vi "Actor Core.vi"(8 "error in":errorcluster, 11 "Measure-Pulse in":refnum<class "Monitor-Pulse.lvclass">) -> (0 "error out":errorcluster, 3 "Actor out":refnum<class "Actor.lvclass">)   [LabVIEW 2016, in "Monitor-Pulse.lvclass"]
doc: "(<B>Filename</B>: Actor Framework.lvlib:Actor.lvclass:Actor Core.vi)\n\nReceives messages to the actor, reacts to them, and initiates any error handling that may shut the actor down.\n\nDescendant classes may override this VI to append parallel tasks for the actor to complete while it handles messages. Overrides use the Call Parent Method node."
uses:
  Monitor-Pulse.lvclass
  C:/github/LabActor/Controllers/Application Controller/Application Controller.lvclass
  C:/github/LabActor/Template Module/Template Module.lvclass
  C:/Program Files/National Instruments/LabVIEW 2016/vi.lib/ActorFramework/Actor/Actor.lvclass
  <vilib>/ActorFramework/Actor/Actor.lvclass
  NHMFL_Core/Libraries/Queued Listbox/Queued Listbox.xctl
  Monitor-Pulse.lvclass/Monitor-Pulse.ctl
  Controllers/Application Controller/Application Controller.lvclass/Application Controller.ctl
  Template Module/Template Module.lvclass/Template Module.ctl
  <vilib>/ActorFramework/Actor/Actor.lvclass/Actor.ctl
  <vilib>/ActorFramework/Message Enqueuer/Message Enqueuer.lvclass/Message Enqueuer.ctl
  Controllers/Application Controller Messages/Pulse Acquired Result/Pulse Acquired Result.lvclass
  C:/github/LabActor/Template Module Messages/Result Reply Msg/Result Reply Msg.lvclass
  Controllers/Application Controller Messages/Pulse Acquired Result/Pulse Acquired Result.lvclass/Pulse Acquired Result.ctl
  Monitor-Pulse Messages/Start Pulse Measurements Msg/Start Measurements Command Msg.lvclass/Start Measurements Command Msg.ctl
  Monitor-Pulse Messages/Stop Measurements Command Msg/Stop Measurements Command Msg.lvclass/Stop Measurements Command Msg.ctl
  <vilib>/Utility/sysdir.llb/System Directory Type.ctl
  Template Module Messages/Save Configuration Msg/Save Configuration Msg.lvclass/Save Configuration Msg.ctl
  Template Module Messages/Open Item Msg/Open Item Msg.lvclass/Open Item Msg.ctl
  Plots/Plot types.ctl
  Controllers/Application Controller Messages/Open Waveform File Plot Msg/Open Waveform File Plot Msg.lvclass/Open Waveform File Plot Msg.ctl
  Controllers/Application Controller Messages/Pulse Acquired Result/Write Open plot.vi
  Controllers/Application Controller/Write Armed ref.vi
  Controllers/Application Controller/Write Monitor Running.vi
  Controllers/Application Controller/Write Monitor ref.vi
  Controllers/Application Controller/Write Postproc ref.vi
  Template Module/Read stop event.vi
  Template Module/Read Open item event.vi
  <vilib>/ActorFramework/Message Enqueuer/Init from Existing Queue.vi
  <vilib>/ActorFramework/Message Enqueuer/Enqueue.vi
  <vilib>/ActorFramework/Stop Msg/Stop Msg.lvclass
  C:/Program Files/National Instruments/LabVIEW 2016/vi.lib/ActorFramework/Message/Message.lvclass
  Monitor-Pulse Messages/Start Pulse Measurements Msg/Start Measurements Command Msg.lvclass
  Monitor-Pulse Messages/Stop Measurements Command Msg/Stop Measurements Command Msg.lvclass
  Template Module Messages/Save Configuration Msg/Save Configuration Msg.lvclass
  Template Module Messages/Open Item Msg/Open Item Msg.lvclass
  Controllers/Application Controller Messages/Open Waveform File Plot Msg/Open Waveform File Plot Msg.lvclass
  <vilib>/ActorFramework/Message Priority Queue/Priority Enqueue.vi
  Controllers/Application Controller/Application Controller.lvclass
  <vilib>/ActorFramework/Message Enqueuer/Message Enqueuer.lvclass
  Template Module Messages/Restore Configuration Msg/Restore Configuration Msg.lvclass
panel:
  in  "Disarm":bool
  in  "Clear log":bool
  out "Error log":string
  in  "Full XY Plot":bool
  out "Monitor file":path caption="Current\nFile"
  in  "View Waveform":bool
  out "PEAK FIELD":dbl format="%#.2g"
  in  "Exit":bool
  in  "Monitor configuration":bool
  in  "Pulse configuration":bool
  in  "Refresh Button":bool
  out "Pulse file":path caption="Last\nFile"
  in  "Write cfg":bool
  in  "Read cfg":bool
  in  "View XY Plot":bool
  out "Monitor Running":bool
  out "Armed":bool
  in  "Arm":bool
  in  "Stop monitor":bool
  in  "Start monitor":bool
  in  "Monitor":string[](xcontrol)
  in  "Process":string[](xcontrol)
  in  "Acquire Pulse":string[](xcontrol)
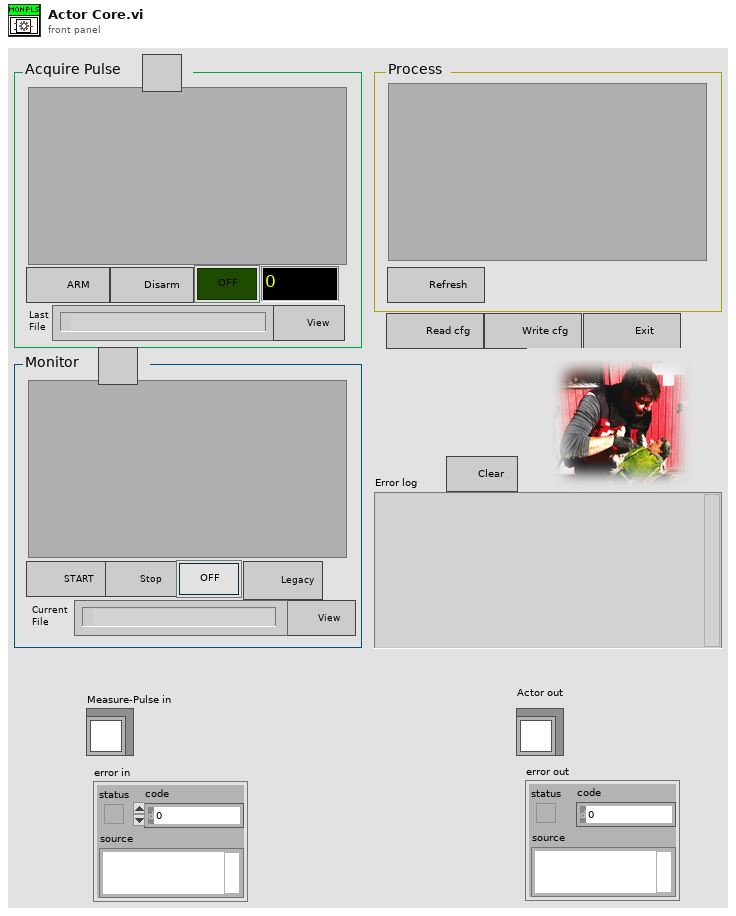
[diagram p1: front panel]
types:
  T1 = typedef "Plot types.ctl" = enum16{"Waveform Plot", "XY Plot", "Full XY"}
  T2 = typedef "System Directory Type.ctl" = i32
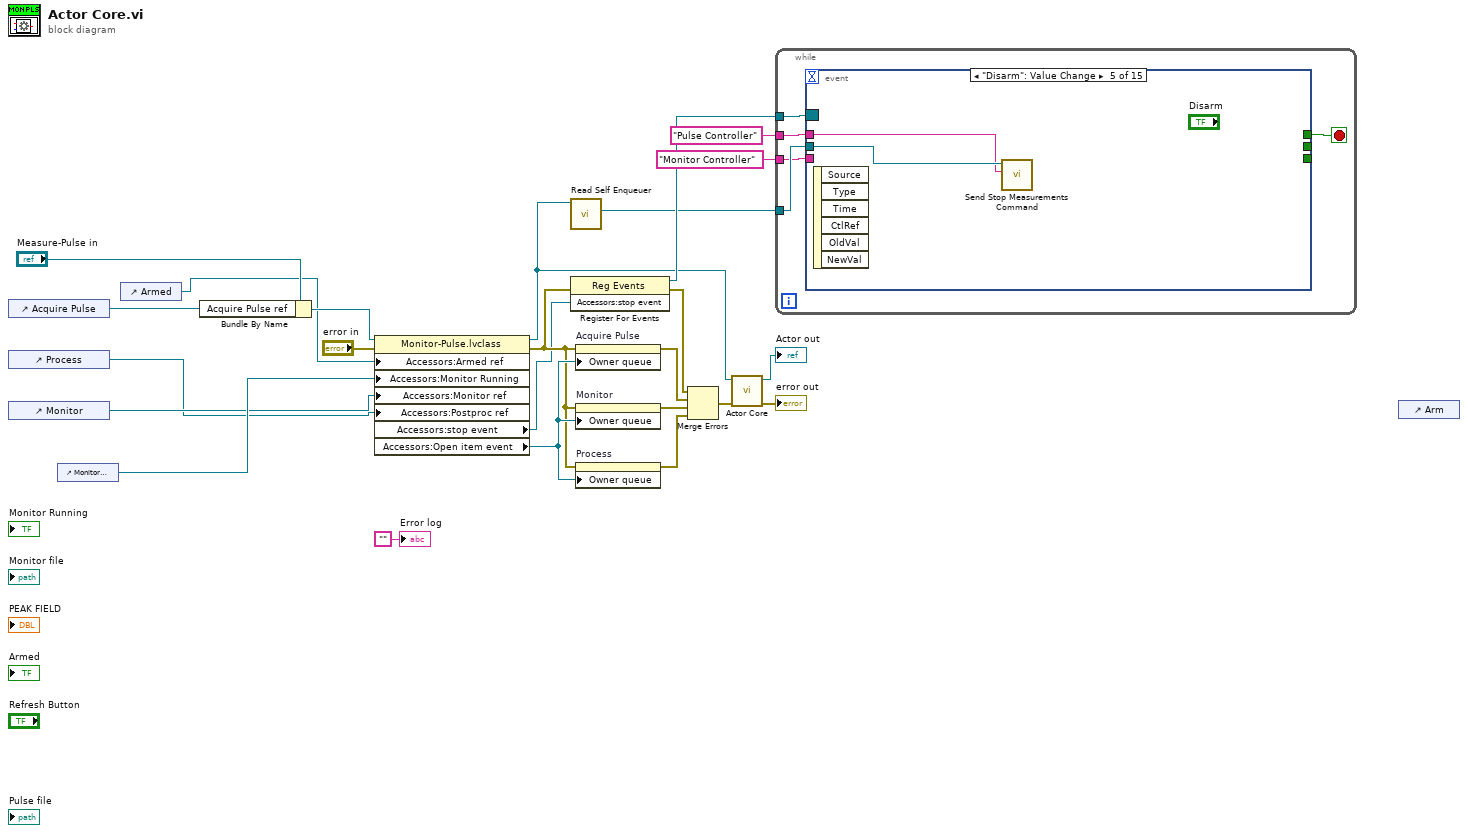
[diagram p0: block diagram]
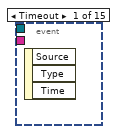
[diagram p2: hidden frame]
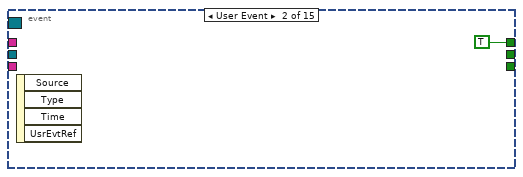
[diagram p3: hidden frame]
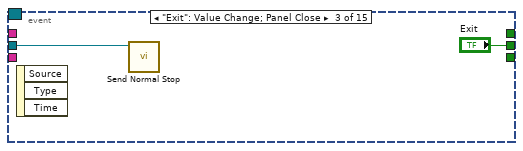
[diagram p4: hidden frame]
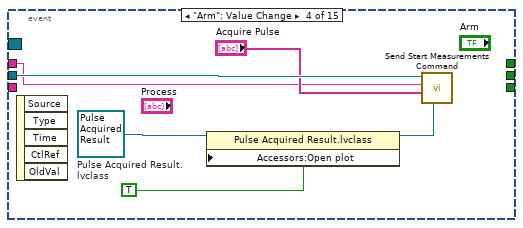
[diagram p5: hidden frame]
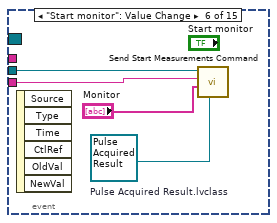
[diagram p6: hidden frame]
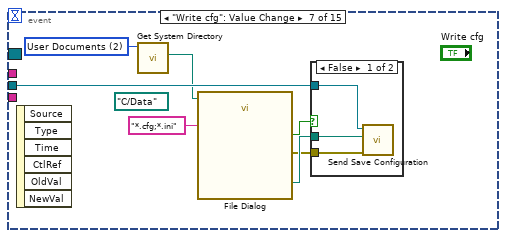
[diagram p7: hidden frame]
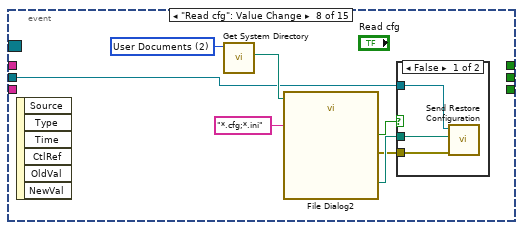
[diagram p9: hidden frame]
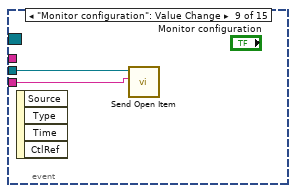
[diagram p11: hidden frame]
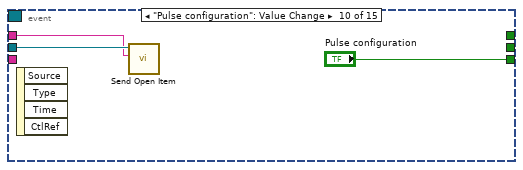
[diagram p12: hidden frame]
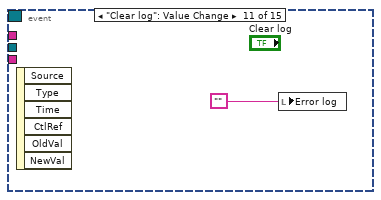
[diagram p13: hidden frame]
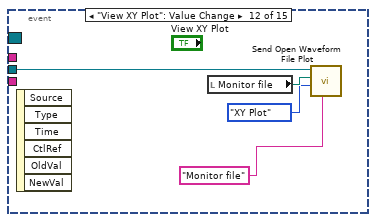
[diagram p14: hidden frame]
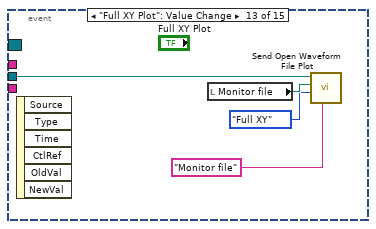
[diagram p15: hidden frame]
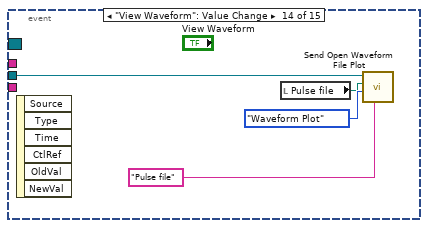
[diagram p16: hidden frame]
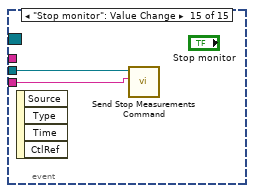
[diagram p17: hidden frame]
diagram:
  n1 = control-ref of="Acquire Pulse"() -> (w9:refnum<vi>)
  n2 = control-ref of="Process"() -> (w1:refnum<vi>)
  n3 = control-ref of="Monitor"() -> (w2:refnum<vi>)
  n4 = control-ref of="Monitor Running"() -> (w3:refnum<vi>)
  n5 = control-ref of="Armed"() -> (w4:refnum<vi>)
  n6 = Bundle By Name(cluster="Measure-Pulse in", "Acquire Pulse ref"=w9) -> (w10:refnum<class "Monitor-Pulse.lvclass">)
  n7 = property class="Monitor-Pulse.lvclass"(reference=w10, error in="error in", "Accessors:Armed ref"=w4, "Accessors:Monitor Running"=w3, "Accessors:Monitor ref"=w2, "Accessors:Postproc ref"=w1) -> (reference out=w12:refnum<class "Monitor-Pulse.lvclass">, error out=w16:errorcluster, "Accessors:stop event"=w5:refnum<user-event>, "Accessors:Open item event"=w20:refnum<user-event>)
  n8 = call <vilib>:"Read Self Enqueuer.vi"("Actor"=w12) -> ("Self Enqueuer"=w11:refnum<class "Message Enqueuer.lvclass">)  [unwired: 10 in]
  n9 = register-events(error in=w16, w5) -> (reference out=w21:refnum<event-registration>, error out=w15:errorcluster)  [unwired: 1 in]
  n10 = property on="Acquire Pulse" class="Queued Listbox (strict)"(error in=w16, "Owner queue"=w20) -> (error out=w19:errorcluster)  [unwired: 1 in, 1 out]
  n11 = property on="Monitor" class="Queued Listbox (strict)"(error in=w16, "Owner queue"=w20) -> (error out=w18:errorcluster)  [unwired: 1 in, 1 out]
  n12 = property on="Process" class="Queued Listbox (strict)"(error in=w16, "Owner queue"=w20) -> (error out=w17:errorcluster)  [unwired: 1 in, 1 out]
  n13 = Merge Errors(w15, w19, w18, w17) -> (w13:errorcluster)
  n14 = call-parent "Actor Core.vi"("error in"=w13, "Measure Object in"=w12) -> ("error out"=→"error out":errorcluster, "Actor out"=→"Actor out":refnum<class "Actor.lvclass">)  [unwired: 8 in]
  n15 = while {
    tunnel: w21 -> [w29]
    tunnel: w11 -> [w27]
    tunnel: "Monitor Controller" ("Controller name") -> [w26]
    tunnel: "Pulse Controller" ("Item name") -> [w25]
    stop <- w28 stop-if-true
    n16 = event shown="[4] \"Disarm\": Value Change" {
      selector: w29 -> [_ _ _ _ _ _ _ _ _ _ _ _ _ _ _]
      dyn-events: _ -> [_ _ _ _ _ _ _ _ _ _ _ _ _ _ _]
      timeout: _ -> [_ _ _ _ _ _ _ _ _ _ _ _ _ _ _]
      tunnel: [_ TRUE _ _ _ _ _ _ _ _ _ _ _ _ _] -> w28
      tunnel: w27 -> [_ _ w31 w38 w40 w43 w48 w56 w66 w68 _ w74 w78 w81 w84]
      tunnel: [_ _ _ _ _ _ _ _ _ "Pulse configuration" _ _ _ _ _] -> _
      tunnel: [_ _ "Exit" _ _ _ _ _ _ _ _ _ _ _ _] -> _
      tunnel: w26 -> [_ _ _ _ _ w42 _ _ w65 _ _ _ _ _ w83]
      tunnel: w25 -> [_ _ _ w36 w39 _ _ _ _ w67 _ _ _ _ _]
      event Timeout {
        n17 = event-data() -> ()  [unwired: 1 in, 3 out]
      }
      event User Event {
        n18 = event-data() -> ()  [unwired: 1 in, 4 out]
      }
      event "Exit": Value Change; Panel Close {
        n19 = event-data() -> ()  [unwired: 1 in, 3 out]
        n20 = call <vilib>:"Send Normal Stop.vi"("Message Enqueuer"=w31) -> ()  [unwired: 10 in, 1 out]
      }
      event "Arm": Value Change {
        w35 = refnum<class "Pulse Acquired Result.lvclass"> refnum  # Pulse Acquired Result.lvclass
        n21 = event-data() -> ()  [unwired: 1 in, 5 out]
        n22 = property class="Pulse Acquired Result.lvclass"(reference=w35, "Accessors:Open plot"=TRUE ("Open plot")) -> (reference out=w34:refnum<class "Pulse Acquired Result.lvclass">)  [unwired: 1 in, 1 out]
        n23 = call "Send Start Measurements Command.vi"("Reply to me"=w34, "Objects"="Acquire Pulse", "Controller name"=w36, "Message Enqueuer"=w38) -> ()  [unwired: 6 in, 2 out]
      }
      event "Disarm": Value Change {
        n24 = event-data() -> ()  [unwired: 1 in, 6 out]
        n25 = call "Send Stop Measurements Command.vi"("Measurement Controller"=w39, "Message Enqueuer"=w40) -> ()  [unwired: 8 in, 2 out]
      }
      event "Start monitor": Value Change {
        w41 = refnum<class "Pulse Acquired Result.lvclass"> refnum  # Pulse Acquired Result.lvclass
        n26 = event-data() -> ()  [unwired: 1 in, 6 out]
        n27 = call "Send Start Measurements Command.vi"("Reply to me"=w41, "Objects"="Monitor", "Controller name"=w42, "Message Enqueuer"=w43) -> ()  [unwired: 6 in, 2 out]
      }
      event "Write cfg": Value Change {
        w46 = T2 2 items=["User Home"=0, "User Desktop"=1, "User Documents"=2, "User Application Data"=3, "User Preferences"=4, "User Temporary"=5, "Public Documents"=6, "Public Application Data"=7, "Public Preferences"=8, "Public Cache"=13, "System Core Libraries"=9, "System Installed Libraries"=10, "Application Files"=11, "Boot Volume Root"=12] ("system directory type")
        (unwired) path "C:/Data" ("start path")
        n28 = event-data() -> ()  [unwired: 1 in, 6 out]
        n29 = call <vilib>:"Get System Directory.vi"("system directory type"=w46) -> ("system directory"=w45:path)  [unwired: 10 in]
        n30 = call "File Dialog"("start path"=w45, "pattern (all files)"="*.cfg;*.ini") -> ("selected path"=w50:path, "cancelled"=w51:bool, "error out"=w47:errorcluster)  [unwired: 10 in, 1 out]
        n31 = case shown="False" w51 {
          tunnel: w50 -> [w52 _]
          tunnel: w48 -> [w54 _]
          tunnel: w47 -> [w53 _]
          frame False {
            n32 = call "Send Save Configuration.vi"("error in (no error)"=w53, "File path"=w52, "Message Enqueuer"=w54) -> ()  [unwired: 7 in, 2 out]
          }
          frame True {
          }
        }
      }
      event "Read cfg": Value Change {
        w58 = T2 2 items=["User Home"=0, "User Desktop"=1, "User Documents"=2, "User Application Data"=3, "User Preferences"=4, "User Temporary"=5, "Public Documents"=6, "Public Application Data"=7, "Public Preferences"=8, "Public Cache"=13, "System Core Libraries"=9, "System Installed Libraries"=10, "Application Files"=11, "Boot Volume Root"=12] ("system directory type")
        n33 = event-data() -> ()  [unwired: 1 in, 6 out]
        n34 = call <vilib>:"Get System Directory.vi"("system directory type"=w58) -> ("system directory"=w57:path)  [unwired: 10 in]
        n35 = call "File Dialog2"("start path"=w57, "pattern (all files)"="*.cfg;*.ini") -> ("selected path"=w61:path, "cancelled"=w55:bool, "error out"=w59:errorcluster)  [unwired: 10 in, 1 out]
        n36 = case shown="False" w55 {
          tunnel: w61 -> [w62 _]
          tunnel: w56 -> [w64 _]
          tunnel: w59 -> [w63 _]
          frame False {
            n37 = call "Send Restore Configuration.vi"("error in (no error)"=w63, "File path"=w62, "Message Enqueuer"=w64) -> ()  [unwired: 7 in, 2 out]
          }
          frame True {
          }
        }
      }
      event "Monitor configuration": Value Change {
        n38 = event-data() -> ()  [unwired: 1 in, 4 out]
        n39 = call "Send Open Item.vi"("Item name"=w65, "Message Enqueuer"=w66) -> ()  [unwired: 8 in, 2 out]
      }
      event "Pulse configuration": Value Change {
        n40 = event-data() -> ()  [unwired: 1 in, 4 out]
        n41 = call "Send Open Item.vi"("Item name"=w67, "Message Enqueuer"=w68) -> ()  [unwired: 8 in, 2 out]
      }
      event "Clear log": Value Change {
        n42 = event-data() -> ()  [unwired: 1 in, 6 out]
        n43 = local write "Error log"("" ("Error log")) -> ()
      }
      event "View XY Plot": Value Change {
        n44 = event-data() -> ()  [unwired: 1 in, 6 out]
        n45 = local read "Monitor file"() -> (w73:path)
        n46 = call "Send Open Waveform File Plot.vi"("Plot group"="Monitor file" ("Control Name"), "Plot type"=Plot_types."XY Plot", "File Path Control"=w73, "Message Enqueuer"=w74) -> ()  [unwired: 6 in, 2 out]
      }
      event "Full XY Plot": Value Change {
        n47 = event-data() -> ()  [unwired: 1 in, 6 out]
        n48 = local read "Monitor file"() -> (w77:path)
        n49 = call "Send Open Waveform File Plot.vi"("Plot group"="Monitor file" ("Control Name"), "Plot type"=Plot_types."Full XY", "File Path Control"=w77, "Message Enqueuer"=w78) -> ()  [unwired: 6 in, 2 out]
      }
      event "View Waveform": Value Change {
        n50 = event-data() -> ()  [unwired: 1 in, 6 out]
        n51 = local read "Pulse file"() -> (w80:path)
        n52 = call "Send Open Waveform File Plot.vi"("Plot group"="Pulse file" ("Control Name"), "Plot type"=Plot_types."Waveform Plot", "File Path Control"=w80, "Message Enqueuer"=w81) -> ()  [unwired: 6 in, 2 out]
      }
      event "Stop monitor": Value Change {
        n53 = event-data() -> ()  [unwired: 1 in, 4 out]
        n54 = call "Send Stop Measurements Command.vi"("Measurement Controller"=w83, "Message Enqueuer"=w84) -> ()  [unwired: 8 in, 2 out]
      }
    }
  }
  n55 = control-ref of="Arm"() -> ()  [unwired: 1 out]
  "Error log" <- "" ("Error log")
